vi "Set_Pulse_Multiple_Channels.vi"(3 "error in":errorcluster, 4 "Pulses":T1[](array[typedef]) {"channel" min=2 max=13 step=1}, 5 "VISA arduino in":refnum<visa-resource-name>) -> (0 "error out":errorcluster, 2 "VISA arduino out":refnum<visa-resource-name>)   [LabVIEW 2021]
uses:
  Channel_Pulse_Stream.ctl
  <vilib>/Utility/error.llb/Error Cluster From Error Code.vi
  <vilib>/ErrorRing/Error Ring.xnode
panel:
  # "Private"
  # "Public"
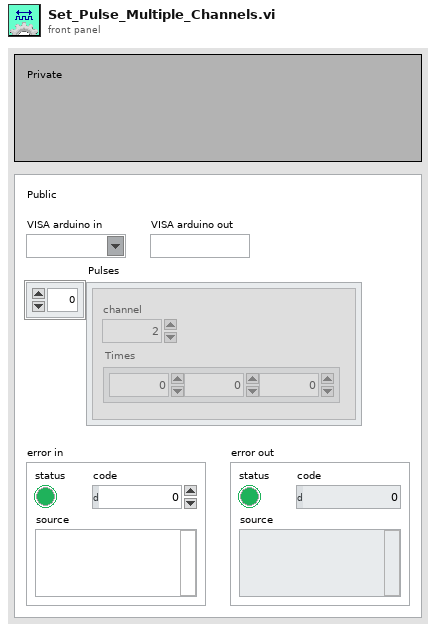
[diagram p1: front panel]
types:
  T1 = typedef "Channel_Pulse_Stream.ctl" = cluster{"Times":dbl[], "channel":u8}
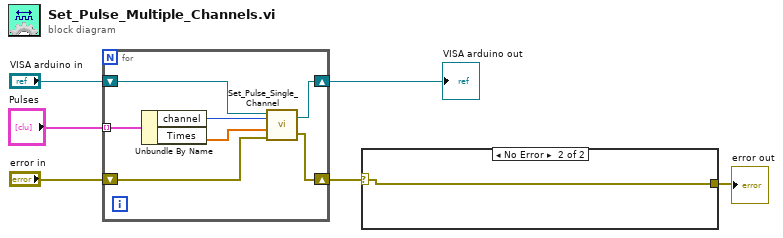
[diagram p0: block diagram]
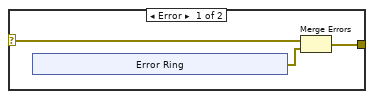
[diagram p2: hidden frame]
diagram:
  n1 = for {
    tunnel: "Pulses" -> [w13] mode=indexing
    shift-right: [w8] -> w2
    shift-left: "error in" -> [w9]
    shift-right: [w7] -> w3
    shift-left: "VISA arduino in" -> [w12]
    n2 = Unbundle By Name(w13) -> ("channel"=w11:u8, "Times"=w10:dbl[])
    n3 = call "Set_Pulse_Single_Channel.vi"("VISA arduino in"=w12, "chanel"=w11, "Times"=w10, "error in"=w9) -> ("VISA arduino out"=w7:refnum<visa-resource-name>, "error out"=w8:errorcluster)  [unwired: 1 in]
  }
  "VISA arduino out" <- w3
  n4 = case shown="No Error" w2 {
    selector: w2 -> [w15 w22]
    tunnel: [w14 w22] -> w1
    frame Error {
      n5 = xnode "Error Ring"() -> ("error out"=w16:errorcluster)
      n6 = Merge Errors(w15, w16) -> (w14:errorcluster)
    }
    frame No Error {
    }
  }
  "error out" <- w1
